vi "Read Packet Type.vi"(8 "error in (no error)":errorcluster, 11 "Packet in":refnum<class "Packet.lvclass">) -> (0 "error out":errorcluster, 2 "Enum":T1, 3 "Packet out":refnum<class "Packet.lvclass">)   [LabVIEW 2019, in "Packet.lvclass"]
uses:
  Packet.lvclass
  packet type STYP.ctl
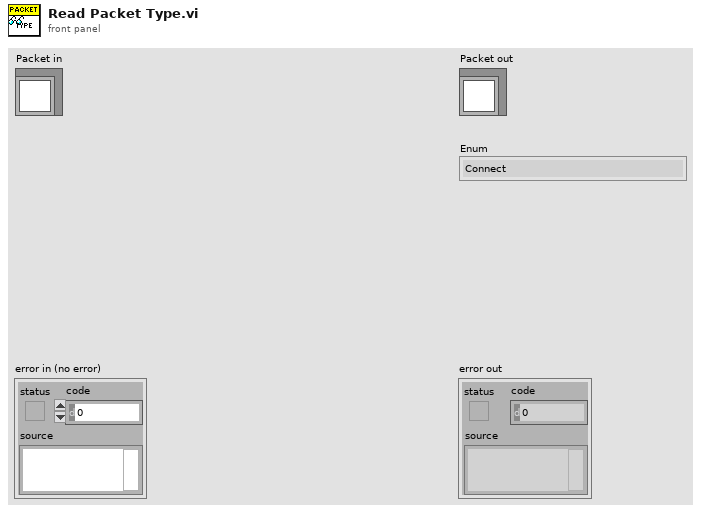
[diagram p1: front panel]
types:
  T1 = typedef "Packet.lvclass/packet type STYP.ctl" = enum16{"Connect", "Disconnect", "Direction", "Score", "Map"}
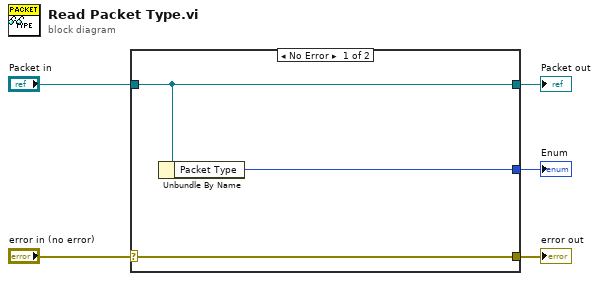
[diagram p0: block diagram]
diagram:
  n1 = case shown="No Error" "error in (no error)" {
    selector: "error in (no error)" -> [w8 w9]
    tunnel: [w8 w9] -> w4
    tunnel: [w7 w10] -> w2
    tunnel: "Packet in" -> [w7 w10]
    tunnel: [w6 _] -> w1
    frame No Error {
      n2 = Unbundle By Name(w7) -> ("Packet Type"=w6:T1)
    }
    frame Error {
    }
  }
  "error out" <- w4
  "Packet out" <- w2
  "Enum" <- w1
